vi "Current Read Array.vi"(8 "error in":errorcluster, 11 "Power Supply In":refnum<class "Power Supply.lvclass">) -> (0 "error out":errorcluster, 1 "Changed or First Call?":bool, 2 "Current SP":dbl[](array[numeric]), 3 "Power Supply Out":refnum<class "Power Supply.lvclass">)   [LabVIEW 2023, in "Power Supply.lvclass"]
uses:
  Power Supply.lvclass
  Power Supply.lvclass/Power Supply.ctl
  Low Level Capabilities/Current/Current Setpoint/Current Setpoint.lvclass
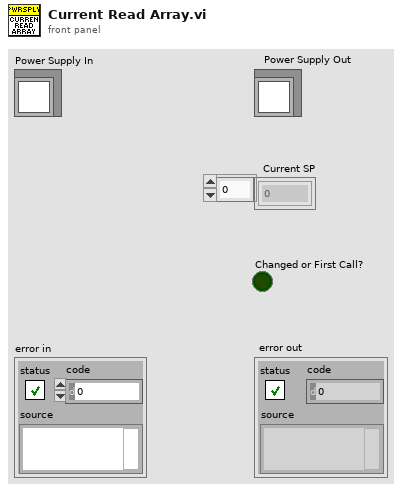
[diagram p1: front panel]
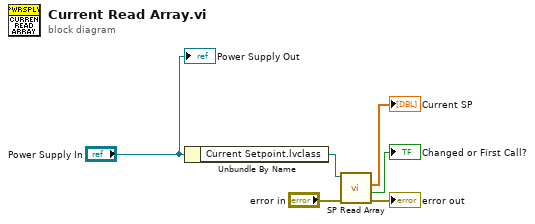
[diagram p0: block diagram]
diagram:
  n1 = Unbundle By Name("Power Supply In") -> ("Current Setpoint.lvclass"=w2:refnum<class "Current Setpoint.lvclass">)
  n2 = call-dynamic "SP Read Array.vi"("error in"="error in", "Current Setpoint in"=w2) -> ("error out"=→"error out":errorcluster, "Changed or First Call?"=→"Changed or First Call?":bool, "Current SP"=→"Current SP":dbl[])  [unwired: 6 in, 1 out]
  "Power Supply Out" <- "Power Supply In"
